vi "Set Value.vi"(8 "error in":errorcluster, 10 "Value":variant, 11 "PDO Mapping Column Header in":refnum<class "PDO Mapping Column Header.lvclass">) -> (0 "error out":errorcluster, 3 "PDO Mapping Column Header out":refnum<class "PDO Mapping Column Header.lvclass">)   [LabVIEW 2019, in "PDO Grid.lvlib" / "PDO Mapping Column Header.lvclass"]
uses:
  PDO Mapping Column Header.lvclass
  Sourcegrid-LabVIEW/source/Cells/ColumnHeader/Column Header.lvclass
  Sourcegrid-LabVIEW/source/Color/Color.lvclass
  Sourcegrid-LabVIEW/source/Views/Cell View/Cell View.lvclass
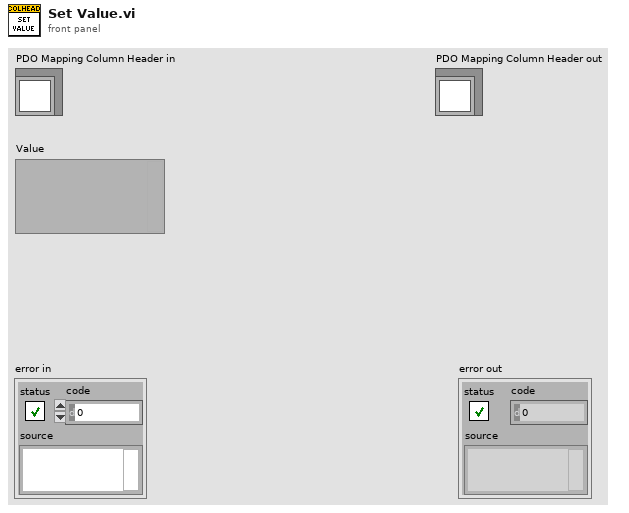
[diagram p1: front panel]
types:
  T1 = enum16{"AliceBlue", "AntiqueWhite", "Aqua", "Aquamarine", "Azure", "Beige", "Bisque", "Black", "BlanchedAlmond", "Blue", "BlueViolet", "Brown", "BurlyWood", "CadetBlue", "Chartreuse", "Chocolate", "Coral", "CornflowerBlue", "Cornsilk", "Crimson", "Cyan", "DarkBlue", "DarkCyan", "DarkGoldenrod", "DarkGray", "DarkGreen", "DarkKhaki", "DarkMagenta", "DarkOliveGreen", "DarkOrange", "DarkOrchid", "DarkRed", "DarkSalmon", "DarkSeaGreen", "DarkSlateBlue", "DarkSlateGray", "DarkTurquoise", "DarkViolet", "DeepPink", "DeepSkyBlue", "DimGray", "DodgerBlue", "Firebrick", "FloralWhite", "ForestGreen", "Fuchsia", "Gainsboro", "GhostWhite", "Gold", "Goldenrod", "Gray", "Green", "GreenYellow", "Honeydew", "HotPink", "IndianRed", "Indigo", "Ivory", "Khaki", "Lavender", "LavenderBlush", "LawnGreen", "LemonChiffon", "LightBlue", "LightCoral", "LightCyan", "LightGoldenrodYellow", "LightGray", "LightGreen", "LightPink", "LightSalmon", "LightSeaGreen", "LightSkyBlue", "LightSlateGray", "LightSteelBlue", "LightYellow", "Lime", "LimeGreen", "Linen", "Magenta", "Maroon", "MediumAquamarine", "MediumBlue", "MediumOrchid", "MediumPurple", "MediumSeaGreen", "MediumSlateBlue", "MediumSpringGreen", "MediumTurquoise", "MediumVioletRed", "MidnightBlue", "MintCream", "MistyRose", "Moccasin", "NavajoWhite", "Navy", "OldLace", "Olive", "OliveDrab", "Orange", "OrangeRed", "Orchid", "PaleGoldenrod", "PaleGreen", "PaleTurquoise", "PaleVioletRed", "PapayaWhip", "PeachPuff", "Peru", "Pink", "Plum", "PowderBlue", "Purple", "Red", "RosyBrown", "RoyalBlue", "SaddleBrown", "Salmon", "SandyBrown", "SeaGreen", "SeaShell", "Sienna", "Silver", "SkyBlue", "SlateBlue", "SlateGray", "Snow", "SpringGreen", "SteelBlue", "Tan", "Teal", "Thistle", "Tomato", "Transparent", "Turquoise", "Violet", "Wheat", "White", "WhiteSmoke", "Yellow"}
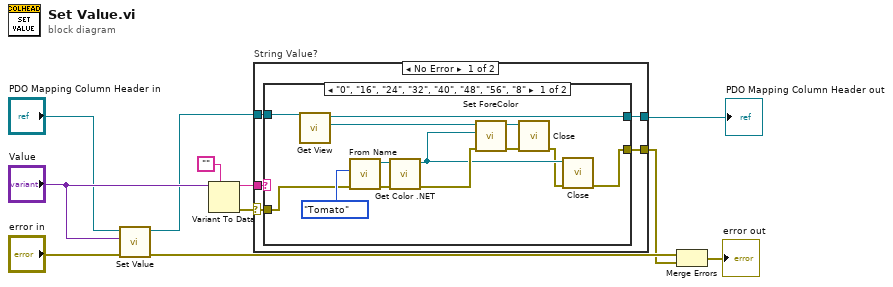
[diagram p0: block diagram]
diagram:
  n1 = call-parent "Set Value.vi"("error in"="error in", "Value"="Value", "Cell in"="PDO Mapping Column Header in") -> ("error out"=w5:errorcluster, "Cell out"=w7:refnum<class "PDO Mapping Column Header.lvclass">)  [unwired: 7 in]
  n2 = Variant To Data(type="", Variant="Value") -> (data=w8:string, error out=w6:errorcluster)  [unwired: 1 in]
  n3 = case "String Value?" shown="No Error" w6 {
    selector: w6 -> [w14 _]
    tunnel: w8 -> [w16 _]
    tunnel: w7 -> [w15 w31]
    tunnel: [w13 w31] -> w1
    tunnel: [w12 _] -> w3
    frame No Error {
      n4 = case shown="\"0\", \"16\", \"24\", \"32\", \"40\", \"48\", \"56\", \"8\"" w16 {
        tunnel: w15 -> [w28 w30]
        tunnel: w14 -> [w25 w29]
        tunnel: [w27 w30] -> w13
        tunnel: [w19 w29] -> w12
        frame "0", "16", "24", "32", "40", "48", "56", "8" {
          n5 = call-dynamic "Get View.vi"("Cell in"=w28) -> ("View"=w23:refnum<class "Cell View.lvclass">, "Cell out"=w27:refnum<class "PDO Mapping Column Header.lvclass">)  [unwired: 8 in, 1 out]
          n6 = call "From Name.vi"("error in"=w25, "Color"=T1."Tomato") -> ("error out"=w22:errorcluster, "Color out"=w24:refnum<class "Color.lvclass">)  [unwired: 8 in]
          n7 = call "Get Color .NET.vi"("Color in"=w24) -> ("Color out"=w21:refnum<class "Color.lvclass">)  [unwired: 9 in, 1 out]
          n8 = call-dynamic "Set ForeColor.vi"("error in"=w22, "Color"=w21, "View in"=w23) -> ("error out"=w20:errorcluster, "View out"=w17:refnum<class "Cell View.lvclass">)  [unwired: 7 in]
          n9 = call-dynamic "Close.vi"("error in"=w20, "Cell View in"=w17) -> ("error out"=w18:errorcluster)  [unwired: 8 in, 1 out]
          n10 = call-dynamic "Close.vi"("error in"=w18, "Color in"=w21) -> ("error out"=w19:errorcluster)  [unwired: 8 in, 1 out]
        }
        frame Default {
        }
      }
    }
    frame Error {
    }
  }
  "PDO Mapping Column Header out" <- w1
  n11 = Merge Errors(w5, w3) -> (→"error out":errorcluster)
